vi "LV SCISDK Set Parameter Double.vi"(8 "error in (no error)":errorcluster, 9 "handle":u64, 10 "value":dbl, 11 "Path":string) -> (0 "error out":errorcluster, 3 "function return":i32)   [LabVIEW 2021, in "SciSDK_Labview.lvlib"]
doc: "SCISDKLABVIEW_DLL_API int LV_SCISDK_SetParameterDouble(char* Path, double value, void* handle);"
uses:
  SciSDK_Labview.lvlib
  <userlib>/SciSDK_Labview/SciSDK_Labview.dll
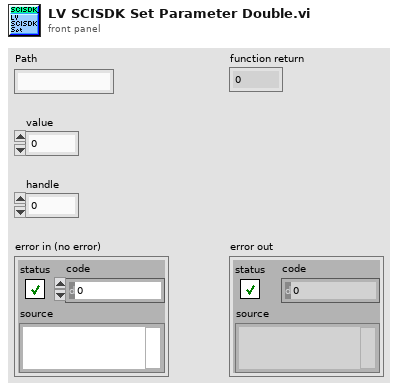
[diagram p1: front panel]
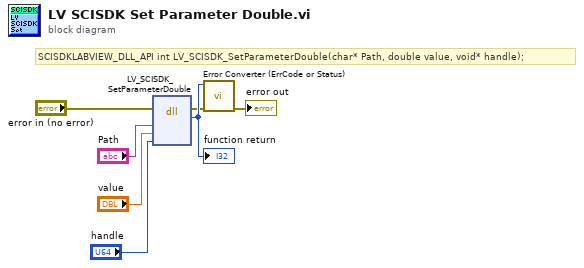
[diagram p0: block diagram]
diagram:
  # "SCISDKLABVIEW_DLL_API int LV_SCISDK_SetParameterDouble(char* Path, double value, void* handle);"
  n1 = dll-call lib="C:/Program Files/National Instruments/LabVIEW 2021/user.lib/SciSDK_Labview/SciSDK_Labview.*" fn="LV_SCISDK_SetParameterDouble"(error in="error in (no error)", "Path"="Path", "value"="value", "handle"="handle") -> (error out=w2:errorcluster, w7:i32)  [unwired: 5 in, 1 out]
  "function return" <- w7
  n2 = call <userlib>:"Error Converter (ErrCode or Status).vi"("error in (no error)"=w2, "error code"=w7) -> ("error out"=→"error out":errorcluster)  [unwired: 9 in]
